vi "Compiled Caller.vi"(0 "x":dbl, 11 "error in":errorcluster) -> (4 "result":dbl, 15 "error out":errorcluster)   [LabVIEW 2026]
doc: "Repro caller: error case, then a Flat Sequence around a project-local Call and a nested Case."
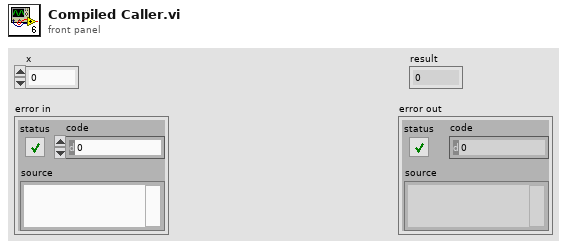
[diagram p1: front panel]
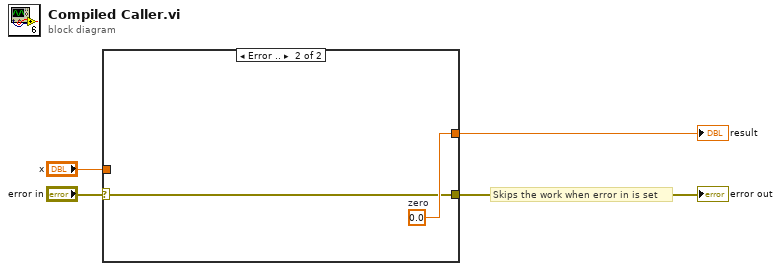
[diagram p0: block diagram]
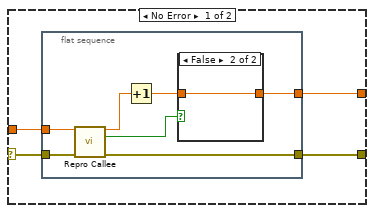
[diagram p2: hidden frame]
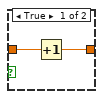
[diagram p3: hidden frame]
diagram:
  # "Skips the work when error in is set"
  n1 = case shown="Error .." "error in" {
    selector: "error in" -> [w5 w19]
    tunnel: "x" -> [w8 _]
    tunnel: [w7 w20] -> w2
    tunnel: [w6 w19] -> w1
    frame No Error {
      n2 = flat-sequence {
        tunnel: w5 -> [w14]
        tunnel: w8 -> [w15]
        tunnel: [w10] -> w7
        tunnel: [w9] -> w6
        frame #0 {
          n3 = call "Repro Callee.vi"("x"=w15, "error in"=w14) -> ("y"=w13:dbl, "positive"=w11:bool, "error out"=w9:errorcluster)  [unwired: 11 in]
          n4 = Increment(x=w13) -> (x+1=w12:dbl)
          n5 = case shown="False" w11 {
            tunnel: w12 -> [w17 w18]
            tunnel: [w16 w18] -> w10
            frame True {
              n6 = Increment(x=w17) -> (x+1=w16:dbl)
            }
            frame False {
            }
          }
        }
      }
    }
    frame Error {
      w20 = 0.0  # zero
    }
  }
  "result" <- w2
  "error out" <- w1
